vi "Config.Check.vi"(8 "error in (no error)":errorcluster, 11 "State Variables":T1={"Events.State"=refnum, "Events.Test Result"=refnum, "Events.Progress"=refnum, "INI.Settings"={"Build Location"=path "C:/Simple Sequence Editor/SequenceRepo", "LoggingLocation"=path "", "Sequence.AbortChannel"="", "Sequence.IterationInfoChannel"="", "Sequence.DurationChannel"="", "Sequence.StepInfoChannel"="", "Sequence.SkipChannel"="", "PlotChannels"=[], "Sequence.InitializeScript"=path "C:/Simple Sequence Editor/SequenceRepo", "Sequence.CleanupScript"=path "", "Log.DefaultRate"=0.0}, "NIVS.AlarmManager"=refnum, "NIVS.BaseLogPath"=path "", "NIVS.DataLogManagerRef"=refnum, "NIVS.DataLogSpecRef"=refnum, "NIVS.Deployed"=FALSE, "NIVS.Events"={"SequenceEvent"=refnum, "SystemChangeEvent"=refnum, "WorkspaceEvent"=refnum}, "NIVS.GatewayIPAddress"="", "NIVS.DataLogGUID"="", "NIVS.ProfileCallback"=refnum, "NIVS.ProfileRef"=refnum, "NIVS.SequenceState"=enum."Idle", "NIVS.SystemDefinitionFile"=path "", "NIVS.SystemStateRefs"={"CustDatRef"=refnum, "EvtRef"=refnum, "Target State User Event"=refnum}, "NIVS.WorkspaceManager"=refnum, "NIVS.EventLogGUID"="", "NIVS.EventLogManagerRef"=refnum, "NIVS.EventLogSpecRef"=refnum, "NIVS.BaseToolPath"=path "", "Restart.Path"=path "", "Sequence.#ofColumns"=0, "Sequence.Iterations"=0, "Sequence.Channels"=[], "Sequence.ValidConfig?"=FALSE, "Station.ID"="", "UDP.Queue"=refnum, "UI.Abort"=refnum, "UI.Alarms"=refnum, "UI.Apply"=refnum, "UI.Back"=refnum, "UI.BaseFileName"=refnum, "UI.CurrentIteration"=refnum, "UI.CurrentStep"=refnum, "UI.CyclicFrequency"=refnum, "UI.Description"=refnum, "UI.DelayTime"=refnum, "UI.DisableAlarms"=refnum, "UI.Duration"=refnum, "UI.EnableLogging"=refnum, "UI.EnableState"=refnum, "UI.High"=refnum, "UI.LogChannels"=refnum, "UI.Low"=refnum, "UI.MonitoredVariable"=refnum, "UI.Next"=refnum, "UI.NumberOfCycles"=refnum, "UI.OperatorName"=refnum, "UI.Pause"=refnum, "UI.Profile"=refnum, "UI.Revert"=refnum, "UI.Skip"=refnum, "UI.Start"=refnum, "UI.StartIteration"=refnum, "UI.StartStep"=refnum, "UI.TabControl"=refnum, "UI.TotalIterations"=refnum, "UI.WaveformDefinition"=refnum, "UI.WaveformPreview"=refnum, "UI.WorkOrderNumber"=refnum, "UI.Chart"=refnum, "UI.Status"=refnum, "UI.DataView"=refnum, "UI.Table"=refnum, "UI.Multihead"=refnum, "UI.ToolTab"=refnum, "UI.Result"=refnum, "UI.Log Path"=refnum, "UI.ReportPath"=refnum, "UI.RestartPath"=refnum, "UI.AlarmLog"=refnum}) -> (0 "error out":errorcluster, 3 "Valid Config?":bool)   [LabVIEW 2015, in "Single Station Execution.lvlib"]
uses:
  Single Station Execution.lvlib
  Types/Main.StateVariables.ctl
  Types/INI.Settings.ctl
  <vilib>/NI Veristand/Execution/AlarmManager/AlarmManagerAPI.ctl
  NationalInstruments.VeriStand.ClientAPI
  <vilib>/NI Veristand/Execution/DataLogging/IDataLogging Ref.ctl
  <vilib>/NI Veristand/Execution/DataLogging/DataLoggingSpecification Ref.ctl
  Types/Execute.UserEventRefs.ctl
  <vilib>/NI Veristand/Execution/Workspace/SystemStateRegEventRef.ctl
  <vilib>/NI Veristand/Execution/Workspace/Target State Info.ctl
  <vilib>/NI Veristand/Execution/Workspace/Target State.ctl
  Types/Execution.SequenceState.ctl
  <vilib>/NI Veristand/Execution/Workspace/SystemStateEventRef.ctl
  <vilib>/NI Veristand/Execution/Workspace/WorkspaceAPI.ctl
  Types/UDPEngine.QueueCluster.ctl
  Types/UDPEngine.State.ctl
  <vilib>/NI Veristand/Execution/Workspace/NI_VS Workspace ExecutionAPI.lvlib
  <vilib>/NI Veristand/Execution/DataLogging/NI_VS Data Logging API.lvlib
  <vilib>/NI Veristand/Execution/AlarmManager/NI_VS AlarmManager ExecutionAPI.lvlib
  NationalInstruments.VeriStand.RealTimeSequenceDefinitionApi
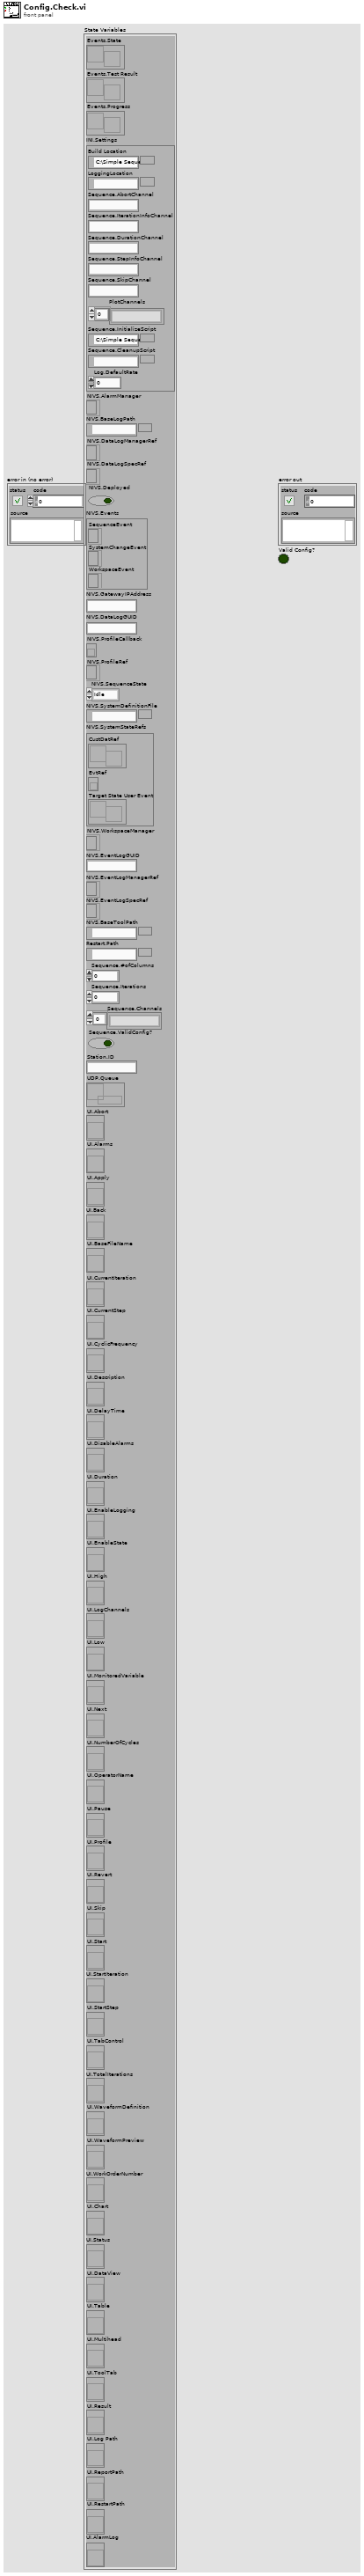
[diagram p1: front panel]
types:
  T1 = typedef "Single Station Execution.lvlib/Main.StateVariables.ctl" = cluster{"Events.State":refnum<user-event>, "Events.Test Result":refnum<user-event>, "Events.Progress":refnum<user-event>, "INI.Settings":T2, "NIVS.AlarmManager":T3, "NIVS.BaseLogPath":path, "NIVS.DataLogManagerRef":T4, "NIVS.DataLogSpecRef":T5, "NIVS.Deployed":bool, "NIVS.Events":T6, "NIVS.GatewayIPAddress":string, "NIVS.DataLogGUID":string, "NIVS.ProfileCallback":refnum<k27>, "NIVS.ProfileRef":refnum<k24>, "NIVS.SequenceState":T8, "NIVS.SystemDefinitionFile":path, "NIVS.SystemStateRefs":T9, "NIVS.WorkspaceManager":T10, "NIVS.EventLogGUID":string, "NIVS.EventLogManagerRef":T4, "NIVS.EventLogSpecRef":T5, "NIVS.BaseToolPath":path, "Restart.Path":path, "Sequence.#ofColumns":i32, "Sequence.Iterations":u32, "Sequence.Channels":string[], "Sequence.ValidConfig?":bool, "Station.ID":string, "UDP.Queue":refnum<queue>, "UI.Abort":refnum<vi>, "UI.Alarms":refnum<vi>, "UI.Apply":refnum<vi>, "UI.Back":refnum<vi>, "UI.BaseFileName":refnum<vi>, "UI.CurrentIteration":refnum<vi>, "UI.CurrentStep":refnum<vi>, "UI.CyclicFrequency":refnum<vi>, "UI.Description":refnum<vi>, "UI.DelayTime":refnum<vi>, "UI.DisableAlarms":refnum<vi>, "UI.Duration":refnum<vi>, "UI.EnableLogging":refnum<vi>, "UI.EnableState":refnum<vi>, "UI.High":refnum<vi>, "UI.LogChannels":refnum<vi>, "UI.Low":refnum<vi>, "UI.MonitoredVariable":refnum<vi>, "UI.Next":refnum<vi>, "UI.NumberOfCycles":refnum<vi>, "UI.OperatorName":refnum<vi>, "UI.Pause":refnum<vi>, "UI.Profile":refnum<vi>, "UI.Revert":refnum<vi>, "UI.Skip":refnum<vi>, "UI.Start":refnum<vi>, "UI.StartIteration":refnum<vi>, "UI.StartStep":refnum<vi>, "UI.TabControl":refnum<vi>, "UI.TotalIterations":refnum<vi>, "UI.WaveformDefinition":refnum<vi>, "UI.WaveformPreview":refnum<vi>, "UI.WorkOrderNumber":refnum<vi>, "UI.Chart":refnum<vi>, "UI.Status":refnum<vi>, "UI.DataView":refnum<vi>, "UI.Table":refnum<vi>, "UI.Multihead":refnum<vi>, "UI.ToolTab":refnum<vi>, "UI.Result":refnum<vi>, "UI.Log Path":refnum<vi>, "UI.ReportPath":refnum<vi>, "UI.RestartPath":refnum<vi>, "UI.AlarmLog":refnum<vi>}
  T2 = typedef "Single Station Execution.lvlib/INI.Settings.ctl" = cluster{"Build Location":path, "LoggingLocation":path, "Sequence.AbortChannel":string, "Sequence.IterationInfoChannel":string, "Sequence.DurationChannel":string, "Sequence.StepInfoChannel":string, "Sequence.SkipChannel":string, "PlotChannels":string[], "Sequence.InitializeScript":path, "Sequence.CleanupScript":path, "Log.DefaultRate":dbl}
  T3 = typedef "NI_VS AlarmManager ExecutionAPI.lvlib/AlarmManagerAPI.ctl" = refnum<k24>
  T4 = typedef "NI_VS Data Logging API.lvlib/IDataLogging Ref.ctl" = refnum<k24>
  T5 = typedef "NI_VS Data Logging API.lvlib/DataLoggingSpecification Ref.ctl" = refnum<k24>
  T6 = typedef "Single Station Execution.lvlib/Execute.UserEventRefs.ctl" = cluster{"SequenceEvent":refnum<event-registration>, "SystemChangeEvent":T7, "WorkspaceEvent":refnum<event-registration>}
  T7 = typedef "NI_VS Workspace ExecutionAPI.lvlib/SystemStateRegEventRef.ctl" = refnum<event-registration>
  T8 = typedef "Single Station Execution.lvlib/Execution.SequenceState.ctl" = enum16{"Idle", "Initializing", "Running", "Paused", "Finalizing", "Complete"}
  T9 = typedef "NI_VS Workspace ExecutionAPI.lvlib/SystemStateEventRef.ctl" = cluster{"CustDatRef":refnum<user-event>, "EvtRef":refnum<k27>, "Target State User Event":refnum<user-event>}
  T10 = typedef "NI_VS Workspace ExecutionAPI.lvlib/WorkspaceAPI.ctl" = refnum<k24>
  T11 = enum8{"Enabled", "Disabled", "Disabled and Grayed Out"}
  T12 = typedef "Single Station Execution.lvlib/Saved.Sequence.ctl" = cluster{"Output Channels":T13[], "Data":dbl[][]}
  T13 = typedef "Single Station Execution.lvlib/Channel.Properties.ctl" = cluster{"Name":string, "NodePath":string, "ScaleUnits":string}
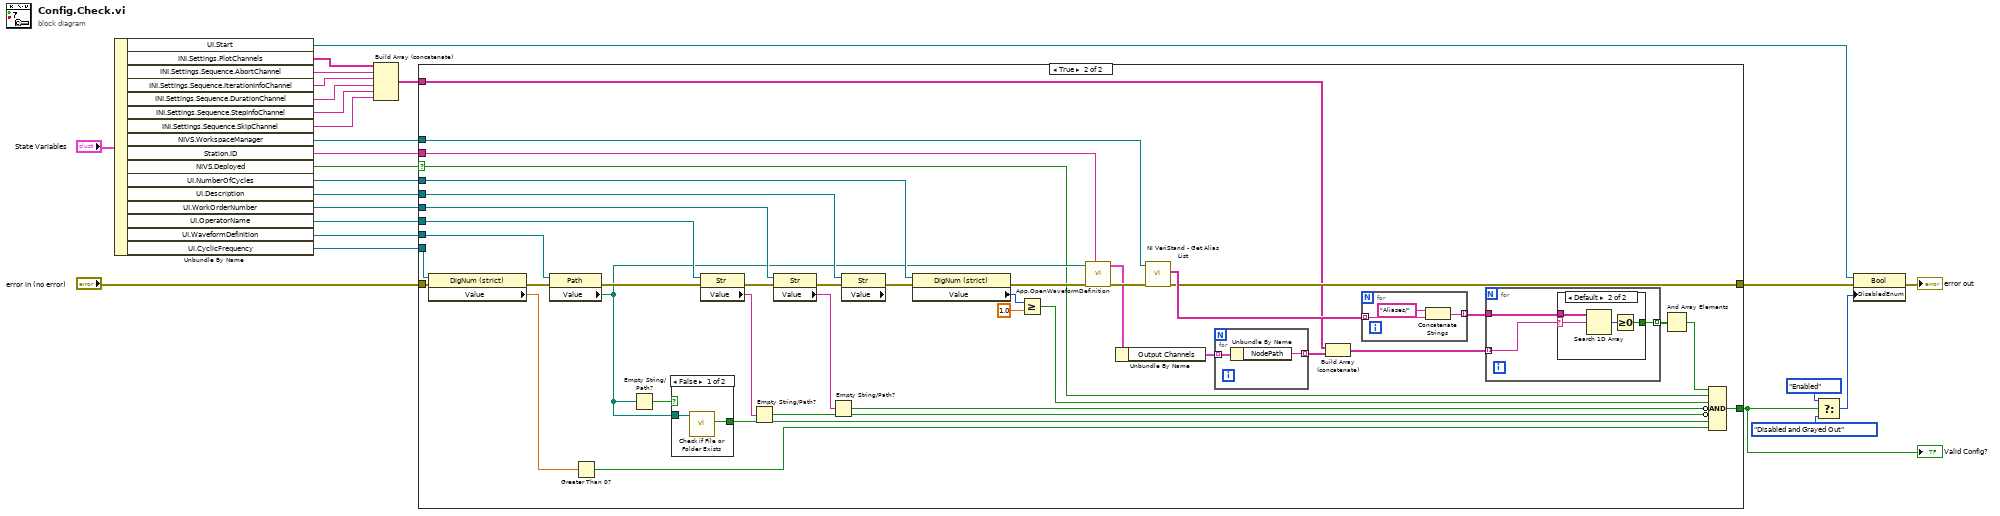
[diagram p0: block diagram]
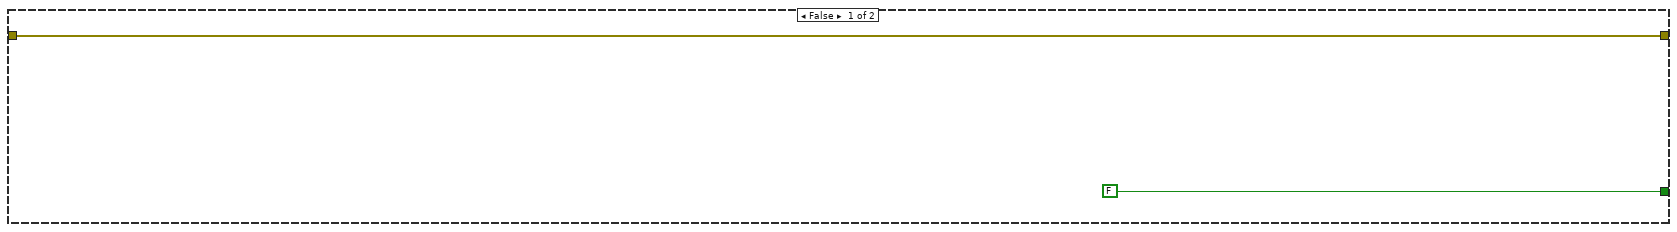
[diagram p2: hidden frame]
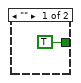
[diagram p4: hidden frame]
diagram:
  n1 = Unbundle By Name("State Variables") -> ("UI.Start"=w17:refnum<vi>, "INI.Settings.PlotChannels"=w1:string[], "INI.Settings.Sequence.AbortChannel"=w8:string, "INI.Settings.Sequence.IterationInfoChannel"=w7:string, "INI.Settings.Sequence.DurationChannel"=w6:string, "INI.Settings.Sequence.StepInfoChannel"=w5:string, "INI.Settings.Sequence.SkipChannel"=w4:string, "NIVS.WorkspaceManager"=w11:T10, "Station.ID"=w2:string, "NIVS.Deployed"=w9:bool, "UI.NumberOfCycles"=w20:refnum<vi>, "UI.Description"=w21:refnum<vi>, "UI.WorkOrderNumber"=w22:refnum<vi>, "UI.OperatorName"=w23:refnum<vi>, "UI.WaveformDefinition"=w24:refnum<vi>, "UI.CyclicFrequency"=w25:refnum<vi>)
  n2 = Build Array (concatenate)(w1, w8, w7, w6, w5, w4) -> (w3:string[])
  n3 = case shown="True" w9 {
    selector: w9 -> [_ w33]
    tunnel: w25 -> [_ w67]
    tunnel: w24 -> [_ w66]
    tunnel: w23 -> [_ w64]
    tunnel: w22 -> [_ w62]
    tunnel: w21 -> [_ w60]
    tunnel: w20 -> [_ w58]
    tunnel: "error in (no error)" -> [w27 w56]
    tunnel: [FALSE w45] -> w12
    tunnel: w11 -> [_ w42]
    tunnel: [w27 w37] -> w10
    tunnel: w3 -> [_ w31]
    tunnel: w2 -> [_ w28]
    frame False {
    }
    frame True {
      n4 = property class="DigNum (strict)"(reference=w67, error in=w56) -> (error out=w65:errorcluster, "Value"=w53:dbl)  [unwired: 1 out]
      n5 = property class="Path"(reference=w66, error in=w65) -> (error out=w63:errorcluster, "Value"=w35:path)  [unwired: 1 out]
      n6 = Greater Than 0?(x=w53) -> (x > 0?=w46:bool)
      n7 = Empty String/Path?(string/path=w35) -> (empty?=w34:bool)
      n8 = case shown="False" w34 {
        tunnel: [w71 _] -> w47
        tunnel: w35 -> [w70 _]
        frame False {
          n9 = call <vilib>:"Check if File or Folder Exists.vi"("path"=w70) -> ("file or folder exists?"=w71:bool)  [unwired: 8 in, 2 out]
        }
        frame True {
        }
      }
      n10 = property class="Str"(reference=w64, error in=w63) -> (error out=w61:errorcluster, "Value"=w52:string)  [unwired: 1 out]
      n11 = Empty String/Path?(string/path=w52) -> (empty?=w49:bool)
      n12 = property class="Str"(reference=w62, error in=w61) -> (error out=w59:errorcluster, "Value"=w51:string)  [unwired: 1 out]
      n13 = Empty String/Path?(string/path=w51) -> (empty?=w48:bool)
      n14 = property class="Str" props=["Value"](reference=w60, error in=w59) -> (error out=w57:errorcluster)  [unwired: 2 out]
      n15 = property class="DigNum (strict)"(reference=w58, error in=w57) -> (error out=w41:errorcluster, "Value"=w55:u32)  [unwired: 1 out]
      n16 = Greater Or Equal?(x=w55, y=1.0) -> (x >= y?=w50:bool)
      n17 = call "App.OpenWaveformDefinition.vi"("StationID"=w28, "error in (no error)"=w41, "selected path"=w35) -> ("error out"=w40:errorcluster, "Settings"=w39:T12)  [unwired: 7 in]
      n18 = Unbundle By Name(w39) -> ("Output Channels"=w32:T13[])
      n19 = call <vilib>:"NI VeriStand - Get Alias List.vi"("error in (no error)"=w40, "WorkspaceManager in"=w42) -> ("error out"=w37:errorcluster, "Aliases"=w44:string[])  [unwired: 6 in, 2 out]
      n20 = for {
        tunnel: w32 -> [w69] mode=indexing
        tunnel: [w68] -> w30 mode=indexing
        n21 = Unbundle By Name(w69) -> ("NodePath"=w68:string)
      }
      n22 = Build Array (concatenate)(w31, w30) -> (w29:string[])
      n23 = for {
        tunnel: w44 -> [w82] mode=indexing
        tunnel: [w80] -> w43 mode=indexing
        n24 = Concatenate Strings("Aliases/", w82) -> (w80:string)
      }
      n25 = for {
        tunnel: w43 -> [w73]
        tunnel: [w74] -> w38 mode=indexing
        tunnel: w29 -> [w72] mode=indexing
        n26 = case shown="Default" w72 {
          selector: w72 -> [_ w76]
          tunnel: [TRUE w78] -> w74
          tunnel: w73 -> [_ w77]
          frame "" {
          }
          frame Default {
            n27 = Search 1D Array(1D array=w77, element=w76) -> (index of element=w79:i32)  [unwired: 1 in]
            n28 = Greater Or Equal To 0?(x=w79) -> (x >= 0?=w78:bool)
          }
        }
      }
      n29 = And Array Elements(Boolean array=w38) -> (logical AND=w36:bool)
      n30 = Compound Arithmetic op=AND(w36, w33, w50, invert w48, invert w49, w47, w46) -> (w45:bool)
    }
  }
  "Valid Config?" <- w12
  n31 = Select(t=T11."Enabled" ("Disabled"), s=w12, f=T11."Disabled and Grayed Out" ("Disabled")) -> (s? t:f=w13:T11)
  n32 = property class="Bool"(reference=w17, error in=w10, "DisabledEnum"=w13) -> (error out=→"error out":errorcluster)  [unwired: 1 out]
